vi "launcher.vi"   [LabVIEW 2024, in "Module 1.lvlib"]
uses:
  Module 1.lvlib
  <extravilib>/ChannelInstances/Event Messenger-t'Channel Messages.lvlib-Message Cluster.ctl'.lvlib
  <extravilib>/ChannelInstances/Event Messenger-t'Channel Messages.lvlib-Message Cluster.ctl'/ChannelOp.ctl
panel:
  # "launcher"
types:
  T1 = typedef "Event Messenger-t'Channel Messages.lvlib-Message Cluster.ctl'.lvlib/ChannelOp.ctl" = enum16{"init", "write", "register", "replicate", "probe"}
  T2 = typedef "Event Messenger-t'Channel Messages.lvlib-Message Cluster.ctl'.lvlib/))Channel.ctl" = refnum<queue>
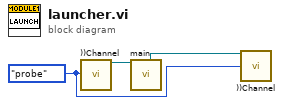
[diagram p0: block diagram]
diagram:
  w1 = ChannelOp."probe" ("channelOp")
  n1 = call <extravilib>:"))Channel.vi"("channelOp"=w1) -> ("channel out"=w3:T2)  [unwired: 10 in, 4 out]
  n2 = call "main.vi"("Message Input"=w3) -> ("Message Output"=w2:T2)  [unwired: 10 in]
  n3 = call <extravilib>:"))Channel.vi"("channel in"=w2, "channelOp"=w1) -> ()  [unwired: 9 in, 5 out]
